vi "Day11-01.vi"() -> ()   [LabVIEW 2021]
uses:
  <vilib>/Instr/_visa.llb/VISA Configure Serial Port (Instr).vi
panel:
  out "온도":u32
  out "문자열":string
  out "Serial Settings:Number of Bytes at Serial Port":u32
  in  "정지":bool
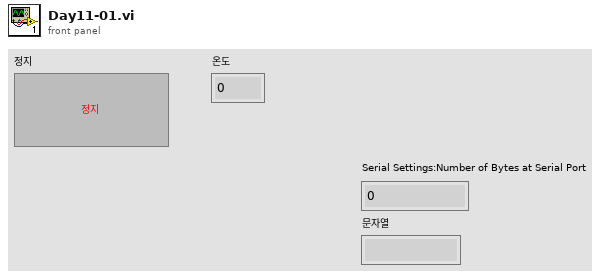
[diagram p1: front panel]
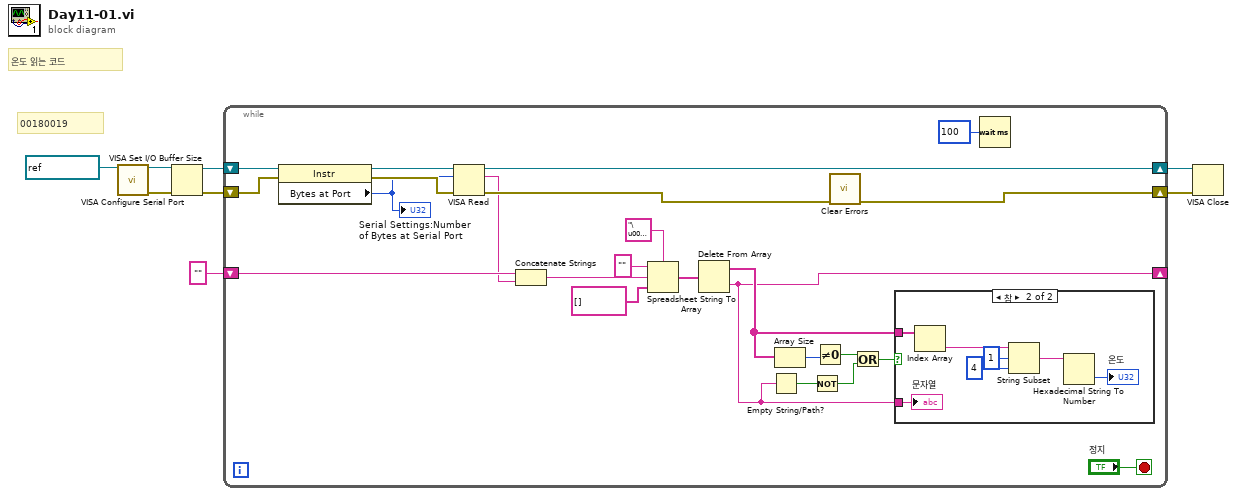
[diagram p0: block diagram]
diagram:
  # "온도 읽는 코드"
  # "00180019"
  n1 = call-poly "VISA Configure Serial Port"("VISA resource name"=refnum<visa-resource-name> "COM5") -> ("VISA resource name out"=w2:refnum<visa-resource-name>, "error out"=w7:errorcluster)  [unwired: 13 in]
  n2 = VISA Set I/O Buffer Size(VISA resource name=w2, error in (no error)=w7) -> (VISA resource name out=w6:refnum<visa-resource-name>, error out=w5:errorcluster)  [unwired: 2 in]
  n3 = while {
    shift-right: [w32] -> w4
    shift-left: w6 -> [w30]
    shift-right: [w9] -> w3
    shift-left: w5 -> [w28]
    shift-right: [w13] -> _
    shift-left: "" ("문자열") -> [w21]
    stop <- "정지" stop-if-true
    n4 = property class="Instr"(reference=w30, error in=w28) -> (reference out=w29:refnum<visa-resource-name>, error out=w27:errorcluster, "Bytes at Port"=w24:u32)
    "Serial Settings:Number of Bytes at Serial Port" <- w24
    n5 = VISA Read(VISA resource name=w29, byte count=w24, error in (no error)=w27) -> (VISA resource name out=w32:refnum<visa-resource-name>, read buffer=w10:string, error out=w31:errorcluster)  [unwired: 1 out]
    n6 = Concatenate Strings(w21, w10) -> (w19:string)
    n7 = Spreadsheet String To Array(delimiter (Tab)="\u0004" ("구분 문자 (탭)"), format string="" ("포맷 문자열"), spreadsheet string=w19, array type (2D Dbl)=string[] []) -> (array=w22:string[])
    n8 = Delete From Array(array=w22) -> (deleted portion=w13:string, array with subset deleted=w16:string[])  [unwired: 2 in]
    n9 = Empty String/Path?(string/path=w13) -> (empty?=w12:bool)
    n10 = Array Size(array=w16) -> (size(s)=w17:i32)
    n11 = Not(x=w12) -> (.not. x?=w11:bool)
    n12 = Not Equal To 0?(x=w17) -> (x != 0?=w15:bool)
    n13 = call <vilib>:"Clear Errors.vi"("error in (no error)"=w31) -> ("error out"=w9:errorcluster)  [unwired: 5 in, 1 out]
    n14 = Or(x=w15, y=w11) -> (x .or. y?=w14:bool)
    n15 = case shown="참" w14 {
      tunnel: w13 -> [_ w39]
      tunnel: w16 -> [_ w38]
      frame False {
      }
      frame True {
        n16 = Index Array(array=w38) -> (element=w37:string)  [unwired: 1 in]
        n17 = String Subset(string=w37, offset (0)=1 ("오프셋(0)"), length (rest)=4 ("길이(나머지)")) -> (substring=w34:string)
        n18 = Hexadecimal String To Number(string=w34) -> (number=→"온도":u32)  [unwired: 2 in, 1 out]
        "문자열" <- w39
      }
    }
    n19 = Wait (ms)(milliseconds to wait=u32 100 ("대기 시간 (ms)")) -> ()  [unwired: 1 out]
  }
  n20 = VISA Close(VISA resource name=w4, error in (no error)=w3) -> ()  [unwired: 1 out]
